vi "okFP Convert Error Code.vi"(8 "error in (no error)":errorcluster, 11 "okFP Error Code":i32) -> (0 "error out":errorcluster)   [LabVIEW 2021, in "okFrontPanelC#Wrapper.lvlib"]
uses:
  okFrontPanelC#Wrapper.lvlib
  okFP Error Codes.ctl
panel:
  in  "okFP Error":T1
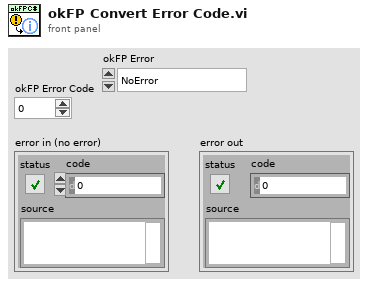
[diagram p1: front panel]
types:
  T1 = typedef "okFrontPanelC#Wrapper.lvlib/okFP Error Codes.ctl" = enum16{"NoError", "Failed", "Timeout", "DoneNotHigh", "TransferError", "CommunicationError", "InvalidBitstream", "FileError", "DeviceNotOpen", "InvalidEndpoint", "InvalidBlockSize", "I2CRestrictedAddress", "I2CBitError", "I2CNack", "I2CUnknownStatus", "UnsupportedFeature", "FIFOUnderflow", "FIFOOverflow", "DataAlignmentError", "InvalidResetProfile", "InvalidParameter"}
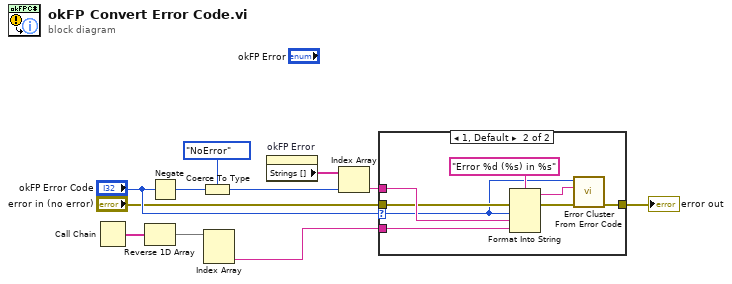
[diagram p0: block diagram]
diagram:
  n1 = Call Chain() -> (call chain=w7:string[])
  n2 = Reverse 1D Array(array=w7) -> (reversed array=w6:string[])
  n3 = Negate(x="okFP Error Code") -> (-x=w11:i32)
  n4 = Coerce To Type(0:w11, 1:okFP_Error_Codes."NoError" ("okFP Error")) -> (2:w8:T1)
  n5 = Index Array(array=w6) -> (element #2=w3:string)  [unwired: 2 in, 1 out]
  n6 = property on="okFP Error" class="Enum (strict)"() -> ("Strings []"=w9:string[])  [unwired: 2 in, 2 out]
  n7 = Index Array(array=w9, index=w8) -> (element=w4:string)
  n8 = case shown="1, Default" "okFP Error Code" {
    selector: "okFP Error Code" -> [_ w14]
    tunnel: w4 -> [_ w19]
    tunnel: w3 -> [_ w18]
    tunnel: "error in (no error)" -> [w12 w17]
    tunnel: [w12 w15] -> w1
    frame 0 {
      # "no error"
    }
    frame 1, Default {
      n9 = Format Into String(format string="Error %d (%s) in %s", error in=w17, w14, w19, w18) -> (resulting string=w13:string, error out=w16:errorcluster)  [unwired: 1 in]
      n10 = call <vilib>:"Error Cluster From Error Code.vi"("error in (no error)"=w16, "error message (\"\")"=w13, "error code (0)"=w14) -> ("error out"=w15:errorcluster)  [unwired: 6 in]
    }
  }
  "error out" <- w1
